vi "DataIn.vi"() -> (7 "AnalogIn0":u16, 8 "AnalogIn1":u16, 9 "AnalogIn2":u16, 10 "AnalogIn3":u16)   [LabVIEW 2020]
uses:
  <vilib>/rvi/Emulation/niFpgaGetClockAttributes.vi
  <vilib>/rvi/Emulation/niFpgaSctlEmulationGetInTimedLoop.vi
  <vilib>/rvi/Emulation/niFpgaEmulationReportErrorSimple.vi
  <vilib>/rvi/eio/common/nirviEmuTemplateMethod_errors.vi
  <vilib>/rvi/Emulation/niFpgaCriticalErrorInLSC.vi
  <vilib>/eio/EIONode/EIONode.xnode
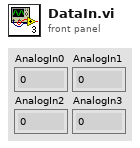
[diagram p1: front panel]
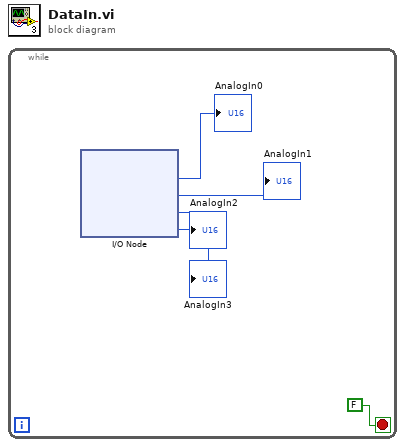
[diagram p0: block diagram]
diagram:
  n1 = while {
    stop <- FALSE stop-if-true
    n2 = xnode "I/O Node"() -> ("AnalogIn0"=→"AnalogIn0":u16, "AnalogIn1"=→"AnalogIn1":u16, "AnalogIn2"=→"AnalogIn2":u16, "AnalogIn3"=→"AnalogIn3":u16)  [unwired: 4 in, 4 out]
  }
